vi "local_normalize.vi"(4 "xmax":dbl, 6 "xmin":dbl, 8 "denoised transmission[r=wl, c=v]":dbl[][](array[numeric]), 9 "voltages in":dbl[](array[numeric])) -> (0 "Locally normalized transmission (r=wl, c=v)":dbl[][](array[numeric]), 1 "Voltages out":dbl[](array[numeric]), 2 "Zeroes (idx)":cluster{"Splice indices":i32[]}[](array[cluster]), 3 "Extrema (type, idx)":T1(array[cluster]), 5 "amplitude graphs":cluster{"Amplitude":cluster{"X":dbl[], dbl[]}}[](array[cluster]), 7 "offset graphs":cluster{"Offset":cluster{"X":dbl[], dbl[]}}[](array[cluster]))   [LabVIEW 2019]
uses:
  REFS.vi
panel:
  in  "Min dist":i32
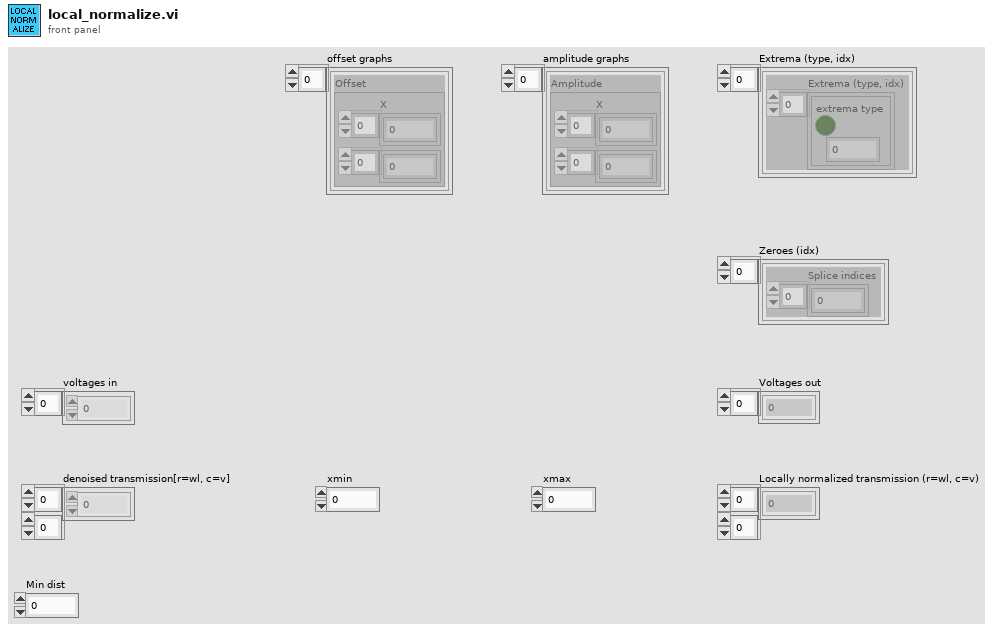
[diagram p1: front panel]
types:
  T1 = cluster{"Extrema (type, idx)":cluster{"extrema type":bool, i32}[]}[]
  T2 = cluster{"Extrema (type, idx)":cluster{"extrema type":bool, i32}[]}
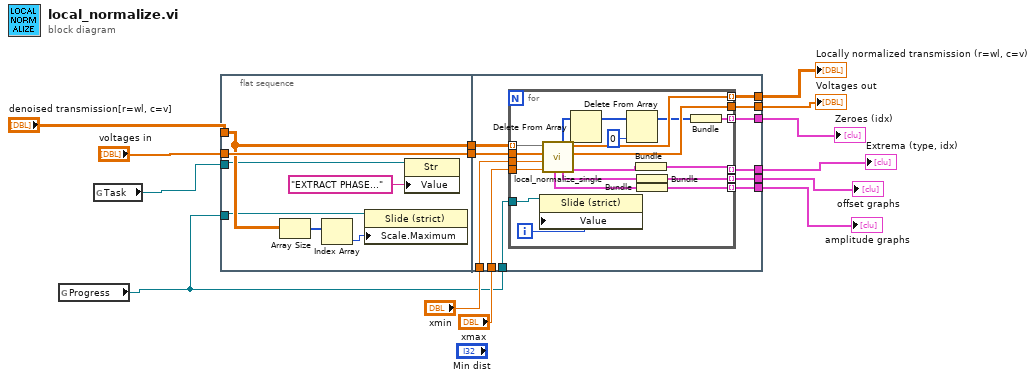
[diagram p0: block diagram]
diagram:
  n1 = global read "REFS.vi" "Progress"() -> (w1:refnum<vi>)
  n2 = global read "REFS.vi" "Task"() -> (w2:refnum<vi>)
  n3 = flat-sequence {
    tunnel: "denoised transmission[r=wl, c=v]" -> [w18]
    tunnel: "voltages in" -> [w21]
    tunnel: [w21] -> w14
    tunnel: [w18] -> w13
    tunnel: w1 -> [w16]
    tunnel: w2 -> [w15]
    tunnel: [w32] -> w9
    tunnel: [w31] -> w10
    tunnel: w14 -> [w30]
    tunnel: w13 -> [w29]
    tunnel: w1 -> [w28]
    tunnel: "xmin" -> [w22]
    tunnel: "xmax" -> [w27]
    tunnel: [w26] -> w7
    tunnel: [w25] -> w6
    tunnel: [w24] -> w3
    tunnel: [w23] -> w5
    frame #0 {
      n4 = Array Size(array=w18) -> (size(s)=w19:i32[])
      n5 = Index Array(array=w19) -> (element=w20:i32)  [unwired: 1 in]
      n6 = property on="Property Node" class="Slide (strict)"(reference=w16, "Scale.Maximum"=w20) -> ()  [unwired: 1 in, 2 out]
      n7 = property class="Str"(reference=w15, "Value"="EXTRACT PHASE...") -> ()  [unwired: 1 in, 2 out]
    }
    frame #1 {
      n8 = for {
        tunnel: w29 -> [w51] mode=indexing
        tunnel: w30 -> [w50]
        tunnel: [w47] -> w32 mode=indexing
        tunnel: [w46] -> w31 mode=indexing
        tunnel: w28 -> [w44]
        tunnel: w22 -> [w43]
        tunnel: w27 -> [w42]
        tunnel: [w41] -> w26 mode=indexing
        tunnel: [w40] -> w25
        tunnel: [w35] -> w24 mode=indexing
        tunnel: [w33] -> w23 mode=indexing
        i -> [w45]
        n9 = property class="Slide (strict)"(reference=w44, "Value"=w45) -> ()  [unwired: 1 in, 2 out]
        n10 = call "local_normalize_single.vi"("xmax"=w42, "xmin"=w43, "X"=w50, "Y"=w51) -> ("Extrema (type, idx)"=w36:cluster{"extrema type":bool, i32}[], "Voltages"=w40:dbl[], "Locally normalized transmission"=w41:dbl[], "Offset"=w48:cluster{"X":dbl[], dbl[]}, "Splice indices"=w39:i32[], "Amplitude"=w49:cluster{"X":dbl[], dbl[]})  [unwired: 2 in]
        n11 = Delete From Array(array=w39) -> (array with subset deleted=w37:i32[])  [unwired: 2 in, 1 out]
        n12 = Delete From Array(array=w37, index=0) -> (array with subset deleted=w34:i32[])  [unwired: 1 in, 1 out]
        n13 = Bundle("Extrema (type, idx)"=w36) -> (w35:T2)  [unwired: 1 in]
        n14 = Bundle("Offset"=w48) -> (w47:cluster{"Offset":cluster{"X":dbl[], dbl[]}})  [unwired: 1 in]
        n15 = Bundle("Amplitude"=w49) -> (w46:cluster{"Amplitude":cluster{"X":dbl[], dbl[]}})  [unwired: 1 in]
        n16 = Bundle("Splice indices"=w34) -> (w33:cluster{"Splice indices":i32[]})  [unwired: 1 in]
      }
    }
  }
  "amplitude graphs" <- w10
  "offset graphs" <- w9
  "Locally normalized transmission (r=wl, c=v)" <- w7
  "Voltages out" <- w6
  "Extrema (type, idx)" <- w3
  "Zeroes (idx)" <- w5
